vi "VI Tree_ND2_Reader_32 bit.vi"   [LabVIEW 2014]
uses:
  controls/cluster_LIMPICTURE.ctl
  controls/cluster_LIMATTRIBUTES.ctl
  <vilib>/vision/Image Controls.llb/IMAQ Image.ctl
  controls/numeric_LIMFILEHANDLE.ctl
  ND2_Reader_32.lvlib
panel:
  # "See Block Diagram"
types:
  T1 = typedef "IMAQ Image.ctl" = refnum<image>
  T2 = typedef "numeric_LIMFILEHANDLE.ctl" = i32
  T3 = typedef "cluster_LIMPICTURE.ctl" = cluster{"uiWidth":u32, "uiHeight":u32, "uiBitsPerComp":u32, "uiComponents":u32, "uiWidthBytes":u32, "uiSize":u32, "pImageData":u32}
  T4 = typedef "cluster_LIMATTRIBUTES.ctl" = cluster{"uiWidth":u32, "uiWidthBytes":u32, "uiHeight":u32, "uiComp":u32, "uiBpcInMemory":u32, "uiBpcSignificant":u32, "uiSequenceCount":u32, "uiTileWidth":u32, "uiTileHeight":u32, "uiCompression":u32, "uiQuality":u16}
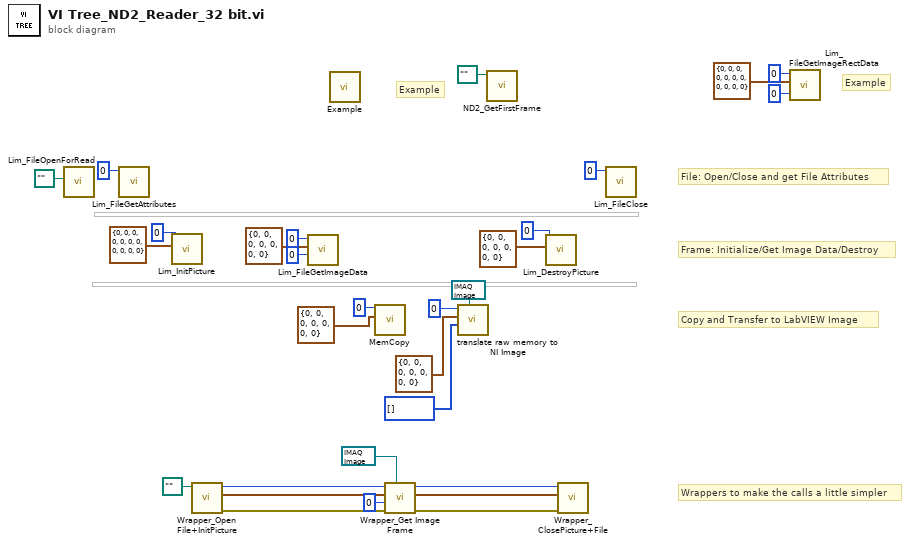
[diagram p0: block diagram]
diagram:
  # "Wrappers to make the calls a little simpler"
  # "Example"
  # "Example"
  # "Copy and Transfer to LabVIEW Image"
  # "Frame: Initialize/Get Image Data/Destroy"
  # "File: Open/Close and get File Attributes"
  n1 = call "Lim_FileOpenForRead.vi"("FilePath"=path "") -> ()  [unwired: 9 in, 2 out]
  n2 = call "Lim_FileGetAttributes.vi"("hFile in"=T2 0) -> ()  [unwired: 6 in, 5 out]
  n3 = call "Lim_InitPicture.vi"("LIMATTRIBUTES"=T4 {"uiWidth"=0, "uiWidthBytes"=0, "uiHeight"=0, "uiComp"=0, "uiBpcInMemory"=0, "uiBpcSignificant"=0, "uiSequenceCount"=0, "uiTileWidth"=0, "uiTileHeight"=0, "uiCompression"=0, "uiQuality"=0}, "hFile in"=T2 0) -> ()  [unwired: 6 in, 4 out]
  n4 = call "Wrapper_Open File+InitPicture.vi"("FilePath"=path "") -> ("error out"=w8:errorcluster, "LIMPICTUREout"=w7:T3, "hFile out"=w9:T2)  [unwired: 7 in, 1 out]
  n5 = call "Lim_FileGetImageData.vi"("frameindex"=u16 0, "LIMPICTURE in"=T3 {"uiWidth"=0, "uiHeight"=0, "uiBitsPerComp"=0, "uiComponents"=0, "uiWidthBytes"=0, "uiSize"=0, "pImageData"=0}, "hFile in"=T2 0) -> ()  [unwired: 5 in, 4 out]
  n6 = call "Example.vi"() -> ()  [unwired: 12 in]
  n7 = call "MemCopy.vi"("LIMPICTURE in"=T3 {"uiWidth"=0, "uiHeight"=0, "uiBitsPerComp"=0, "uiComponents"=0, "uiWidthBytes"=0, "uiSize"=0, "pImageData"=0}, "hFile in"=T2 0) -> ()  [unwired: 6 in, 4 out]
  n8 = call "Wrapper_Get Image Frame.vi"("Image Ref in"=T1 refnum, "error in (no error)"=w8, "frameindex in"=0, "LIMPICTURE in"=w7, "hFile in"=w9) -> ("error out"=w4:errorcluster, "LIMPICTURE out"=w5:T3, "hFile out"=w6:T2)  [unwired: 2 in, 2 out]
  n9 = call "translate raw memory to NI Image.vi"("Image in"=T1 refnum, "pBuffer"=u8[] [], "LIMPICTURE in"=T3 {"uiWidth"=0, "uiHeight"=0, "uiBitsPerComp"=0, "uiComponents"=0, "uiWidthBytes"=0, "uiSize"=0, "pImageData"=0} ("LIMPICTURE out"), "hFile in"=T2 0) -> ()  [unwired: 4 in, 4 out]
  n10 = call "ND2_GetFirstFrame.vi"("FilePath"=path "") -> ()  [unwired: 8 in, 3 out]
  n11 = call "Lim_DestroyPicture.vi"("LIMPICTURE"=T3 {"uiWidth"=0, "uiHeight"=0, "uiBitsPerComp"=0, "uiComponents"=0, "uiWidthBytes"=0, "uiSize"=0, "pImageData"=0}, "hFile in"=T2 0) -> ()  [unwired: 8 in, 2 out]
  n12 = call "Wrapper_ClosePicture+File.vi"("error in (no error)"=w4, "LIMPICTURE"=w5, "hFile in"=w6) -> ()  [unwired: 8 in, 1 out]
  n13 = call "Lim_FileClose.vi"("hFile in"=T2 0) -> ()  [unwired: 9 in, 2 out]
  n14 = call "Lim_FileGetImageRectData.vi"("frameindex"=u32 0, "LIMATTRIBUTES"=T4 {"uiWidth"=0, "uiWidthBytes"=0, "uiHeight"=0, "uiComp"=0, "uiBpcInMemory"=0, "uiBpcSignificant"=0, "uiSequenceCount"=0, "uiTileWidth"=0, "uiTileHeight"=0, "uiCompression"=0, "uiQuality"=0}, "hFile in"=T2 0) -> ()  [unwired: 6 in, 3 out]
